vi "Configuration Parse.vi"(0 "UI Controls":T8 {"measurement configuration"."Low Reference Level (%)" min=0.0 max=100.0 step=1.0; "measurement configuration"."Window Step Size (%)" format="%#_6p"; "measurement configuration"."Window Stop (%)" format="%#_6p"; "measurement configuration"."Measurement Offset" format="%.2p"; "measurement configuration"."Pulse Acquisition Length (s)" format="%.2f"; "measurement configuration"."Pulse Power Level (dBm)" format="%.6p"; "measurement configuration"."Number of Pulses per Burst" format="%#_6p"; "measurement configuration"."Pulse Width (s)" format="%.2f"; "measurement configuration"."Pulse Repetition Interval [PRI] (s)" format="%.3p"; "measurement configuration"."RFSG Generation IQ Rate (S/s)" format="%.3p"; "measurement configuration"."RFmx Reference Level (dBm)" format="%.6p"; "measurement configuration"."RFmx Measurement Bandwidth (Hz)" format="%.3p"; "measurement configuration"."RFmx Center Frequency (Hz)" format="%.6p"; "measurement configuration"."RFmx external attenuation (dB)" format="%.2f"; "measurement configuration"."RFSG external attenuation (dB)" format="%.2f"}, 11 "error in":errorcluster) -> (4 "RFmx Settings":T1={"Center Frequency (Hz)"=10000000000.0, "Measurement Bandwidth (Hz)"=80000000.0, "Reference Level (dBm)"=10.0, "RFmx De-embedding"={"RFmx Name"="5842_0", "RFmx Port"="", "Attenuation"={"Mode"=enum."Constant Attenuation", "Constant Attenuation"={"RFmx External Attenuation (dB)"=1.2}, "s2p File"={"RFmx S-Parameters Orientation"=24000, "RFmx Attenuation s2p Path Name"="", "RFmx Attenuation s2p File"=path ""}}}, "Acquisition Length (s)"=0.0} {"RFmx De-embedding"."Attenuation"."s2p File"."RFmx S-Parameters Orientation" items=["Port1 Towards DUT"=24000, "Port2 Towards DUT"=24001]; "RFmx De-embedding"."Attenuation"."Constant Attenuation"."RFmx External Attenuation (dB)" format="%.2f"; "Reference Level (dBm)" format="%.2f"; "Measurement Bandwidth (Hz)" format="%.3p"; "Center Frequency (Hz)" format="%.6p"}, 6 "RFSG settings":T3={"RFSG De-embedding"={"RFSG Name"="5842_0", "RFSG Port"="", "Attenuation"={"Mode"=enum."Constant Attenuation", "Contant Attenuation"={"RFSG External Attenuation (dB)"=2.0}, "s2p File"={"RFSG S-parameters Orientation"=24000, "RFSG Attenuation s2p Path Name"="", "RFSG s2p File Path"=path ""}}}, "Generation IQ Rate (S/s)"=0.0} {"RFSG De-embedding"."Attenuation"."s2p File"."RFSG S-parameters Orientation" items=["Port1 Towards DUT"=24000, "Port2 Towards DUT"=24001]; "RFSG De-embedding"."Attenuation"."Contant Attenuation"."RFSG External Attenuation (dB)" format="%.2f"}, 8 "Test Configuration":T5, 15 "error out":errorcluster)   [LabVIEW 2023, in "FPT Pulse Measurement.lvclass"]
uses:
  FPT Pulse Measurement.lvclass
  Measurement Configuration.ctl
  Measurement Results.ctl
  Measurement/Controls/Test Config - Pulse.ctl
  Measurement/Controls/RFSG Config - Pulse.ctl
  FPT Shared VIs/De-embedding/RFsg Config.ctl
  Measurement/Controls/RFmx Config - Pulse.ctl
  FPT Shared VIs/De-embedding/RFmx Config.ctl
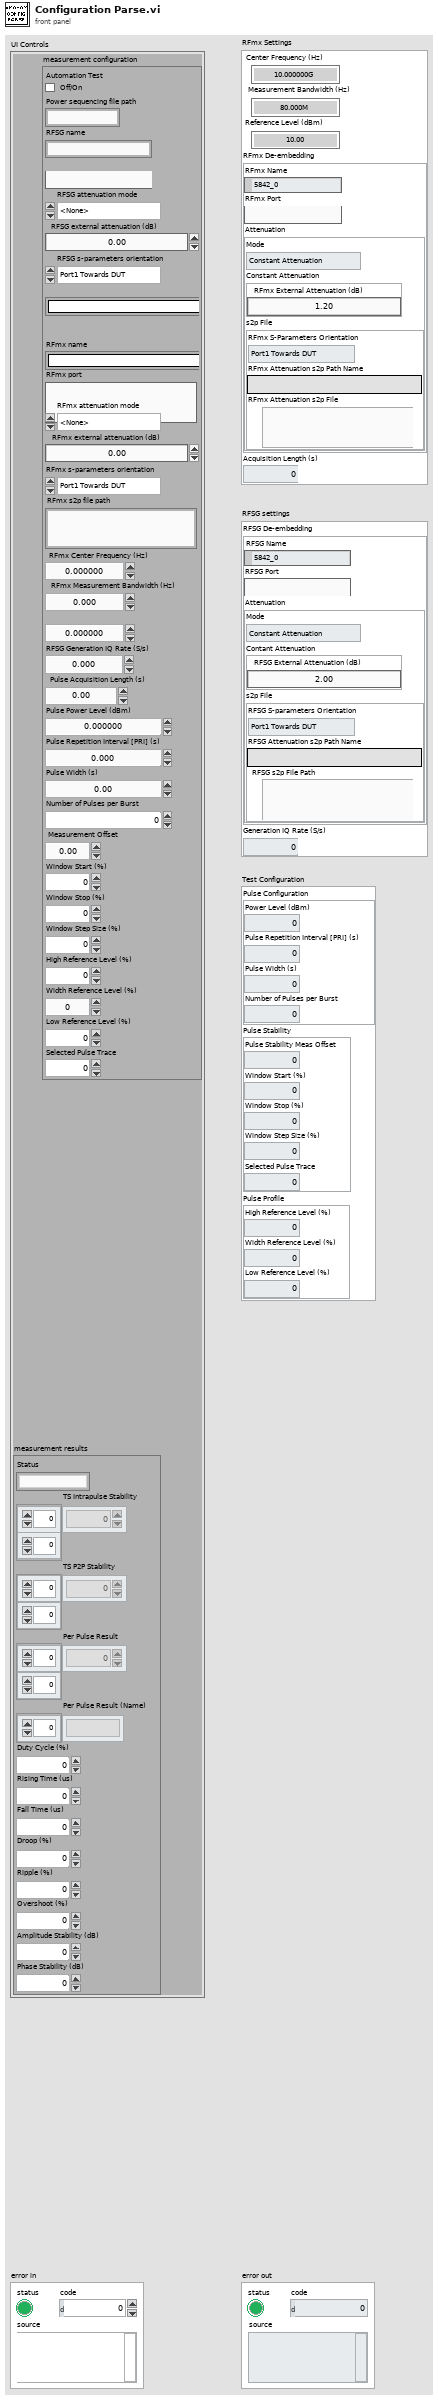
[diagram p1: front panel]
types:
  T1 = typedef "RFmx Config - Pulse.ctl" = cluster{"Center Frequency (Hz)":dbl, "Measurement Bandwidth (Hz)":dbl, "Reference Level (dBm)":dbl, "RFmx De-embedding":T2, "Acquisition Length (s)":dbl}
  T2 = typedef "RFmx Config.ctl" = cluster{"RFmx Name":refnum<k15>, "RFmx Port":string, "Attenuation":cluster{"Mode":enum32{"<None>", "Constant Attenuation", "s2p File"}, "Constant Attenuation":cluster{"RFmx External Attenuation (dB)":dbl}, "s2p File":cluster{"RFmx S-Parameters Orientation":i32, "RFmx Attenuation s2p Path Name":string, "RFmx Attenuation s2p File":path}}}
  T3 = typedef "RFSG Config - Pulse.ctl" = cluster{"RFSG De-embedding":T4, "Generation IQ Rate (S/s)":dbl}
  T4 = typedef "RFsg Config.ctl" = cluster{"RFSG Name":refnum<k15>, "RFSG Port":string, "Attenuation":cluster{"Mode":enum32{"<None>", "Constant Attenuation", "s2p File"}, "Contant Attenuation":cluster{"RFSG External Attenuation (dB)":dbl}, "s2p File":cluster{"RFSG S-parameters Orientation":i32, "RFSG Attenuation s2p Path Name":string, "RFSG s2p File Path":path}}}
  T5 = typedef "Test Config - Pulse.ctl" = cluster{"Pulse Configuration":cluster{"Power Level (dBm)":dbl, "Pulse Repetition Interval [PRI] (s)":dbl, "Pulse Width (s)":dbl, "Number of Pulses per Burst":u32}, "Pulse Stability":cluster{"Pulse Stability Meas Offset":i32, "Window Start (%)":dbl, "Window Stop (%)":dbl, "Window Step Size (%)":dbl, "Selected Pulse Trace":i32}, "Pulse Profile":cluster{"High Reference Level (%)":dbl, "Width Reference Level (%)":dbl, "Low Reference Level (%)":dbl}}
  T6 = typedef "FPT Pulse Measurement.lvclass/Measurement Configuration.ctl" = cluster{"Automation Test":bool, "Power sequencing file path":string, "RFSG name":string, "RFSG port":string, "RFSG attenuation mode":enum32{"<None>", "Constant Attenuation", "s2p File"}, "RFSG external attenuation (dB)":dbl, "RFSG s-parameters orientation":enum32{"Port1 Towards DUT", "Port2 Towards DUT"}, "RFSG s2p file path":string, "RFmx name":string, "RFmx port":string, "RFmx attenuation mode":enum32{"<None>", "Constant Attenuation", "s2p File"}, "RFmx external attenuation (dB)":dbl, "RFmx s-parameters orientation":enum32{"Port1 Towards DUT", "Port2 Towards DUT"}, "RFmx s2p file path":string, "RFmx Center Frequency (Hz)":dbl, "RFmx Measurement Bandwidth (Hz)":dbl, "RFmx Reference Level (dBm)":dbl, "RFSG Generation IQ Rate (S/s)":dbl, "Pulse Acquisition Length (s)":dbl, "Pulse Power Level (dBm)":dbl, "Pulse Repetition Interval [PRI] (s)":dbl, "Pulse Width (s)":dbl, "Number of Pulses per Burst":u32, "Measurement Offset":i32, "Window Start (%)":dbl, "Window Stop (%)":dbl, "Window Step Size (%)":dbl, "High Reference Level (%)":dbl, "Width Reference Level (%)":dbl, "Low Reference Level (%)":dbl, "Selected Pulse Trace":i32}
  T7 = typedef "FPT Pulse Measurement.lvclass/Measurement Results.ctl" = cluster{"Status":string, "TS Intrapulse Stability":dbl[][], "TS P2P Stability":dbl[][], "Per Pulse Result":dbl[][], "Per Pulse Result (Name)":string[], "Duty Cycle (%)":dbl, "Rising Time (us)":dbl, "Fall Time (us)":dbl, "Droop (%)":dbl, "Ripple (%)":dbl, "Overshoot (%)":dbl, "Amplitude Stability (dB)":dbl, "Phase Stability (dB)":dbl}
  T8 = cluster{"measurement configuration":T6, "measurement results":T7}
  T9 = enum32{"<None>", "Constant Attenuation", "s2p File"}
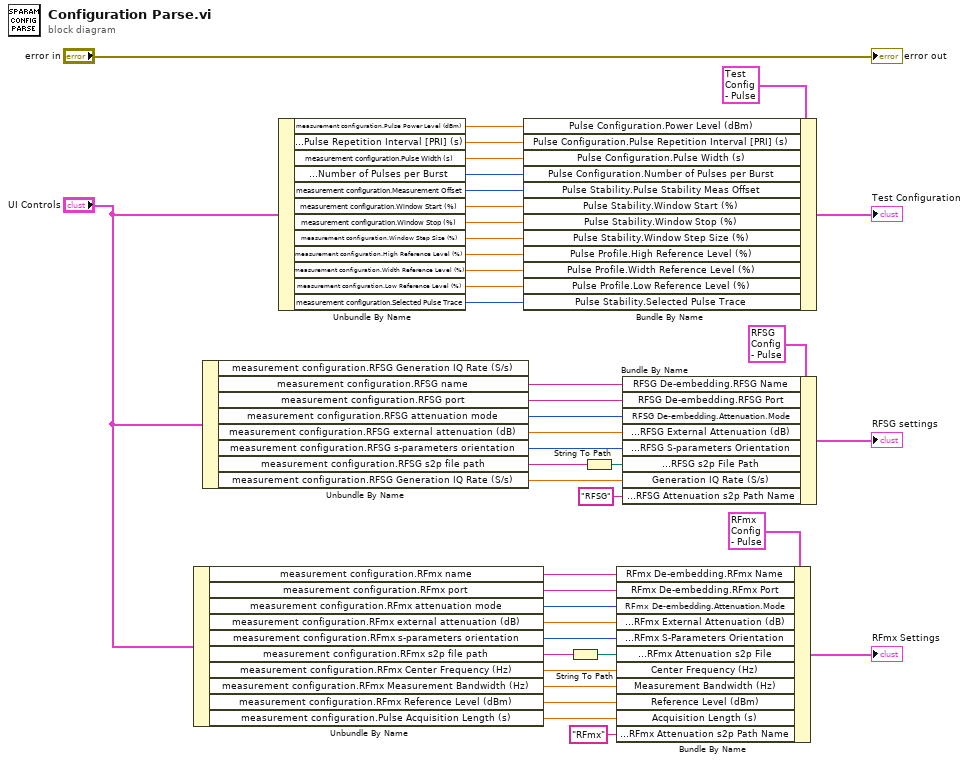
[diagram p0: block diagram]
diagram:
  n1 = Unbundle By Name("UI Controls") -> ("measurement configuration.RFmx name"=w18:string, "measurement configuration.RFmx port"=w19:string, "measurement configuration.RFmx attenuation mode"=w24:T9, "measurement configuration.RFmx external attenuation (dB)"=w23:dbl, "measurement configuration.RFmx s-parameters orientation"=w22:enum32{"Port1 Towards DUT", "Port2 Towards DUT"}, "measurement configuration.RFmx s2p file path"=w20:string, "measurement configuration.RFmx Center Frequency (Hz)"=w8:dbl, "measurement configuration.RFmx Measurement Bandwidth (Hz)"=w7:dbl, "measurement configuration.RFmx Reference Level (dBm)"=w6:dbl, "measurement configuration.Pulse Acquisition Length (s)"=w5:dbl)
  n2 = Unbundle By Name("UI Controls") -> ("measurement configuration.RFSG name"=w16:string, "measurement configuration.RFSG port"=w15:string, "measurement configuration.RFSG attenuation mode"=w29:T9, "measurement configuration.RFSG external attenuation (dB)"=w28:dbl, "measurement configuration.RFSG s-parameters orientation"=w27:enum32{"Port1 Towards DUT", "Port2 Towards DUT"}, "measurement configuration.RFSG s2p file path"=w26:string, "measurement configuration.RFSG Generation IQ Rate (S/s)"=w11:dbl)  [unwired: 1 out]
  n3 = Unbundle By Name("UI Controls") -> ("measurement configuration.Pulse Power Level (dBm)"=w40:dbl, "measurement configuration.Pulse Repetition Interval [PRI] (s)"=w39:dbl, "measurement configuration.Pulse Width (s)"=w38:dbl, "measurement configuration.Number of Pulses per Burst"=w37:u32, "measurement configuration.Measurement Offset"=w36:i32, "measurement configuration.Window Start (%)"=w35:dbl, "measurement configuration.Window Stop (%)"=w34:dbl, "measurement configuration.Window Step Size (%)"=w33:dbl, "measurement configuration.High Reference Level (%)"=w32:dbl, "measurement configuration.Width Reference Level (%)"=w31:dbl, "measurement configuration.Low Reference Level (%)"=w30:dbl, "measurement configuration.Selected Pulse Trace"=w1:i32)
  n4 = Bundle By Name(cluster=T5 {"Pulse Configuration"={"Power Level (dBm)"=0.0, "Pulse Repetition Interval [PRI] (s)"=0.0, "Pulse Width (s)"=0.0, "Number of Pulses per Burst"=0}, "Pulse Stability"={"Pulse Stability Meas Offset"=0, "Window Start (%)"=0.0, "Window Stop (%)"=0.0, "Window Step Size (%)"=0.0, "Selected Pulse Trace"=0}, "Pulse Profile"={"High Reference Level (%)"=0.0, "Width Reference Level (%)"=0.0, "Low Reference Level (%)"=0.0}} ("Test Configuration"), "Pulse Configuration.Power Level (dBm)"=w40, "Pulse Configuration.Pulse Repetition Interval [PRI] (s)"=w39, "Pulse Configuration.Pulse Width (s)"=w38, "Pulse Configuration.Number of Pulses per Burst"=w37, "Pulse Stability.Pulse Stability Meas Offset"=w36, "Pulse Stability.Window Start (%)"=w35, "Pulse Stability.Window Stop (%)"=w34, "Pulse Stability.Window Step Size (%)"=w33, "Pulse Profile.High Reference Level (%)"=w32, "Pulse Profile.Width Reference Level (%)"=w31, "Pulse Profile.Low Reference Level (%)"=w30, "Pulse Stability.Selected Pulse Trace"=w1) -> (→"Test Configuration":T5)
  n5 = String To Path(string=w20) -> (path=w21:path)
  n6 = String To Path(string=w26) -> (path=w25:path)
  n7 = Bundle By Name(cluster=T1 {"Center Frequency (Hz)"=10000000000.0, "Measurement Bandwidth (Hz)"=80000000.0, "Reference Level (dBm)"=10.0, "RFmx De-embedding"={"RFmx Name"="5842_0", "RFmx Port"="", "Attenuation"={"Mode"=enum."Constant Attenuation", "Constant Attenuation"={"RFmx External Attenuation (dB)"=1.2}, "s2p File"={"RFmx S-Parameters Orientation"=24000, "RFmx Attenuation s2p Path Name"="", "RFmx Attenuation s2p File"=path ""}}}, "Acquisition Length (s)"=0.0} ("RFmx Settings"), "RFmx De-embedding.RFmx Name"=w18, "RFmx De-embedding.RFmx Port"=w19, "RFmx De-embedding.Attenuation.Mode"=w24, "RFmx De-embedding.Attenuation.Constant Attenuation.RFmx External Attenuation (dB)"=w23, "RFmx De-embedding.Attenuation.s2p File.RFmx S-Parameters Orientation"=w22, "RFmx De-embedding.Attenuation.s2p File.RFmx Attenuation s2p File"=w21, "Center Frequency (Hz)"=w8, "Measurement Bandwidth (Hz)"=w7, "Reference Level (dBm)"=w6, "Acquisition Length (s)"=w5, "RFmx De-embedding.Attenuation.s2p File.RFmx Attenuation s2p Path Name"="RFmx") -> (→"RFmx Settings":T1)
  n8 = Bundle By Name(cluster=T3 {"RFSG De-embedding"={"RFSG Name"="5842_0", "RFSG Port"="", "Attenuation"={"Mode"=enum."Constant Attenuation", "Contant Attenuation"={"RFSG External Attenuation (dB)"=2.0}, "s2p File"={"RFSG S-parameters Orientation"=24000, "RFSG Attenuation s2p Path Name"="", "RFSG s2p File Path"=path ""}}}, "Generation IQ Rate (S/s)"=0.0} ("RFSG settings"), "RFSG De-embedding.RFSG Name"=w16, "RFSG De-embedding.RFSG Port"=w15, "RFSG De-embedding.Attenuation.Mode"=w29, "RFSG De-embedding.Attenuation.Contant Attenuation.RFSG External Attenuation (dB)"=w28, "RFSG De-embedding.Attenuation.s2p File.RFSG S-parameters Orientation"=w27, "RFSG De-embedding.Attenuation.s2p File.RFSG s2p File Path"=w25, "Generation IQ Rate (S/s)"=w11, "RFSG De-embedding.Attenuation.s2p File.RFSG Attenuation s2p Path Name"="RFSG") -> (→"RFSG settings":T3)
  "error out" <- "error in"
